vi "Histogram2D2011.vi"   [LabVIEW 2013]
uses:
  <vilib>/Heliosphere Research LLC/Advanced Plotting Toolkit/api_plotting/Histogram2DRange.ctl
  ModeType.ctl
  <vilib>/Heliosphere Research LLC/Advanced Plotting Toolkit/api_plotting/Histogram2D_Automatic.vi
  <vilib>/Heliosphere Research LLC/Advanced Plotting Toolkit/Advanced Plotting Toolkit.lvlib
types:
  T1 = typedef "ModeType.ctl" = enum16{"Normal", "Expected Failure", "Skipped"}
  T2 = typedef "Advanced Plotting Toolkit.lvlib/Histogram2DRange.ctl" = cluster{"X Min":dbl, "X Max":dbl, "Y Min":dbl, "Y Max":dbl}
  T3 = typedef "Advanced Plotting Toolkit.lvlib/PlotID.ctl" = i32
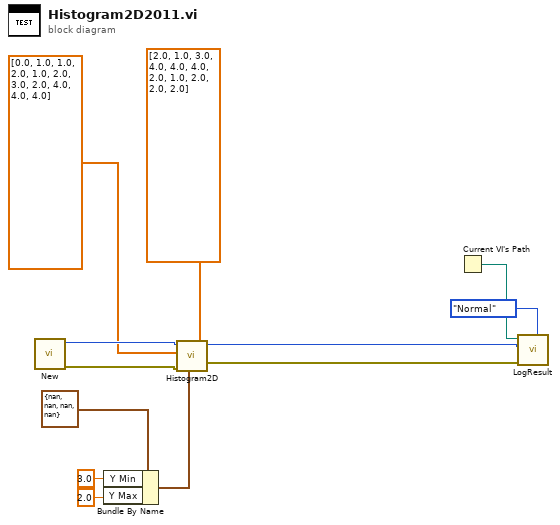
[diagram p0: block diagram]
diagram:
  n1 = call <vilib>:"New.vi"() -> ("error out"=w10:errorcluster, "Plot ID"=w11:T3)  [unwired: 10 in]
  n2 = Bundle By Name(cluster=T2 {"X Min"=nan, "X Max"=nan, "Y Min"=nan, "Y Max"=nan} ("Data Range"), "Y Min"=3.0 ("X Min"), "Y Max"=2.0 ("X Max")) -> (w4:T2)
  n3 = call-poly <vilib>:"Histogram2D.vi"("Data Range"=w4, "error in (no error)"=w10, "Y Data"=dbl[] [2.0, 1.0, 3.0, 4.0, 4.0, 4.0, 2.0, 1.0, 2.0, 2.0, 2.0] ("X Data"), "X Data"=dbl[] [0.0, 1.0, 1.0, 2.0, 1.0, 2.0, 3.0, 2.0, 4.0, 4.0, 4.0], "Plot ID"=w11) -> ("error out"=w8:errorcluster, "Plot ID Out"=w9:T3)  [unwired: 5 in]
  n4 = Current VI's Path() -> (path=w12:path)
  n5 = call "LogResult.vi"("Mode"=ModeType."Normal", "Test Result"=w8, "Test Artifact"=w9, "VI Path"=w12) -> ()  [unwired: 8 in]
